vi "ScrumCollection.vi"() -> ()   [LabVIEW 2016]
panel:
  in  "Tab Control":T1(tab)
  out "Summed Signal":dynamicdata(graph)
  out "Maximum Force":dbl
  in  "Tab Control 2":enum32{"Data Collection", "Settings"}(tab)
  out "Collecting?":bool
  in  "Start/Stop Collection":bool
  in  "Reset Graphs":bool
  in  "Pause datastream":bool=TRUE caption="Enable"
  in  "Load Cell 7":bool
  in  "Load Cell 6":bool
  in  "Load Cell 5":bool
  in  "Load Cell 4":bool
  in  "Load Cell 3":bool
  in  "Load Cell 2":bool
  in  "Load Cell 1":bool
  in  "Load Cell 0":bool
  in  "Are you collecting data?":bool
  out "Collected Section":dynamicdata(graph) caption="Section"
  out "Mean Value for last 20 sec":dbl format="%#.6g"
  in  "Load Cell Offset":dbl
  out "Cell 1":dynamicdata(graph)
  out "Cell 0":dynamicdata(graph)
  in  "Load Cell Offset 1":dbl
  out "Mean Value for last 20 sec 1":dbl format="%#.6g"
  out "Cell 2":dynamicdata(graph)
  out "Cell 3":dynamicdata(graph)
  in  "Load Cell Offset 2":dbl
  in  "Load Cell Offset 3":dbl
  out "Mean Value for last 20 sec 2":dbl format="%#.6g"
  out "Mean Value for last 20 sec 3":dbl format="%#.6g"
  out "Cell 4":dynamicdata(graph)
  out "Cell 5":dynamicdata(graph)
  in  "Load Cell Offset 4":dbl
  in  "Load Cell Offset 5":dbl
  out "Mean Value for last 20 sec 4":dbl format="%#.6g"
  out "Mean Value for last 20 sec 5":dbl format="%#.6g"
  out "Cell 6":dynamicdata(graph)
  out "Cell 7":dynamicdata(graph)
  in  "Load Cell Offset 6":dbl
  in  "Load Cell Offset 7":dbl
  out "Mean Value for last 20 sec 6":dbl format="%#.6g"
  out "Mean Value for last 20 sec 7":dbl format="%#.6g"
  out "Balance":dbl(knob) scale=-2000.0..2000.0
  in  "stop":bool
  # "Which load cells should be included in the main graph?"
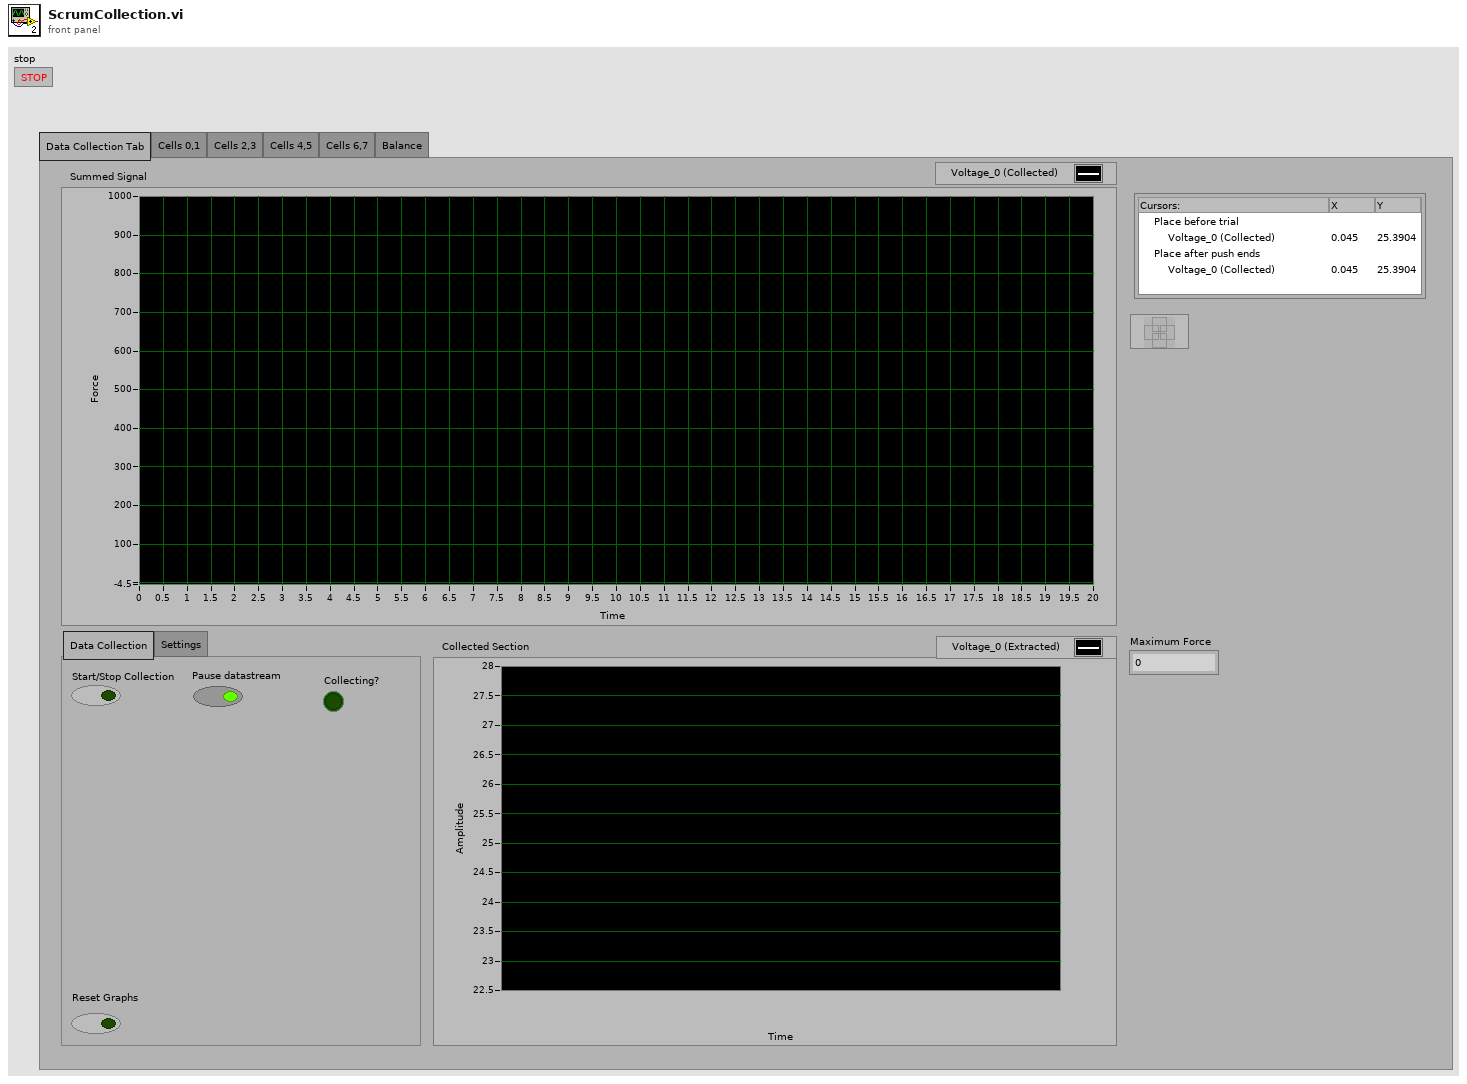
[diagram p1: front panel]
types:
  T1 = enum32{"Data Collection Tab", "Cells 0,1", "Cells 2,3", "Cells 4,5", "Cells 6,7", "Balance"}
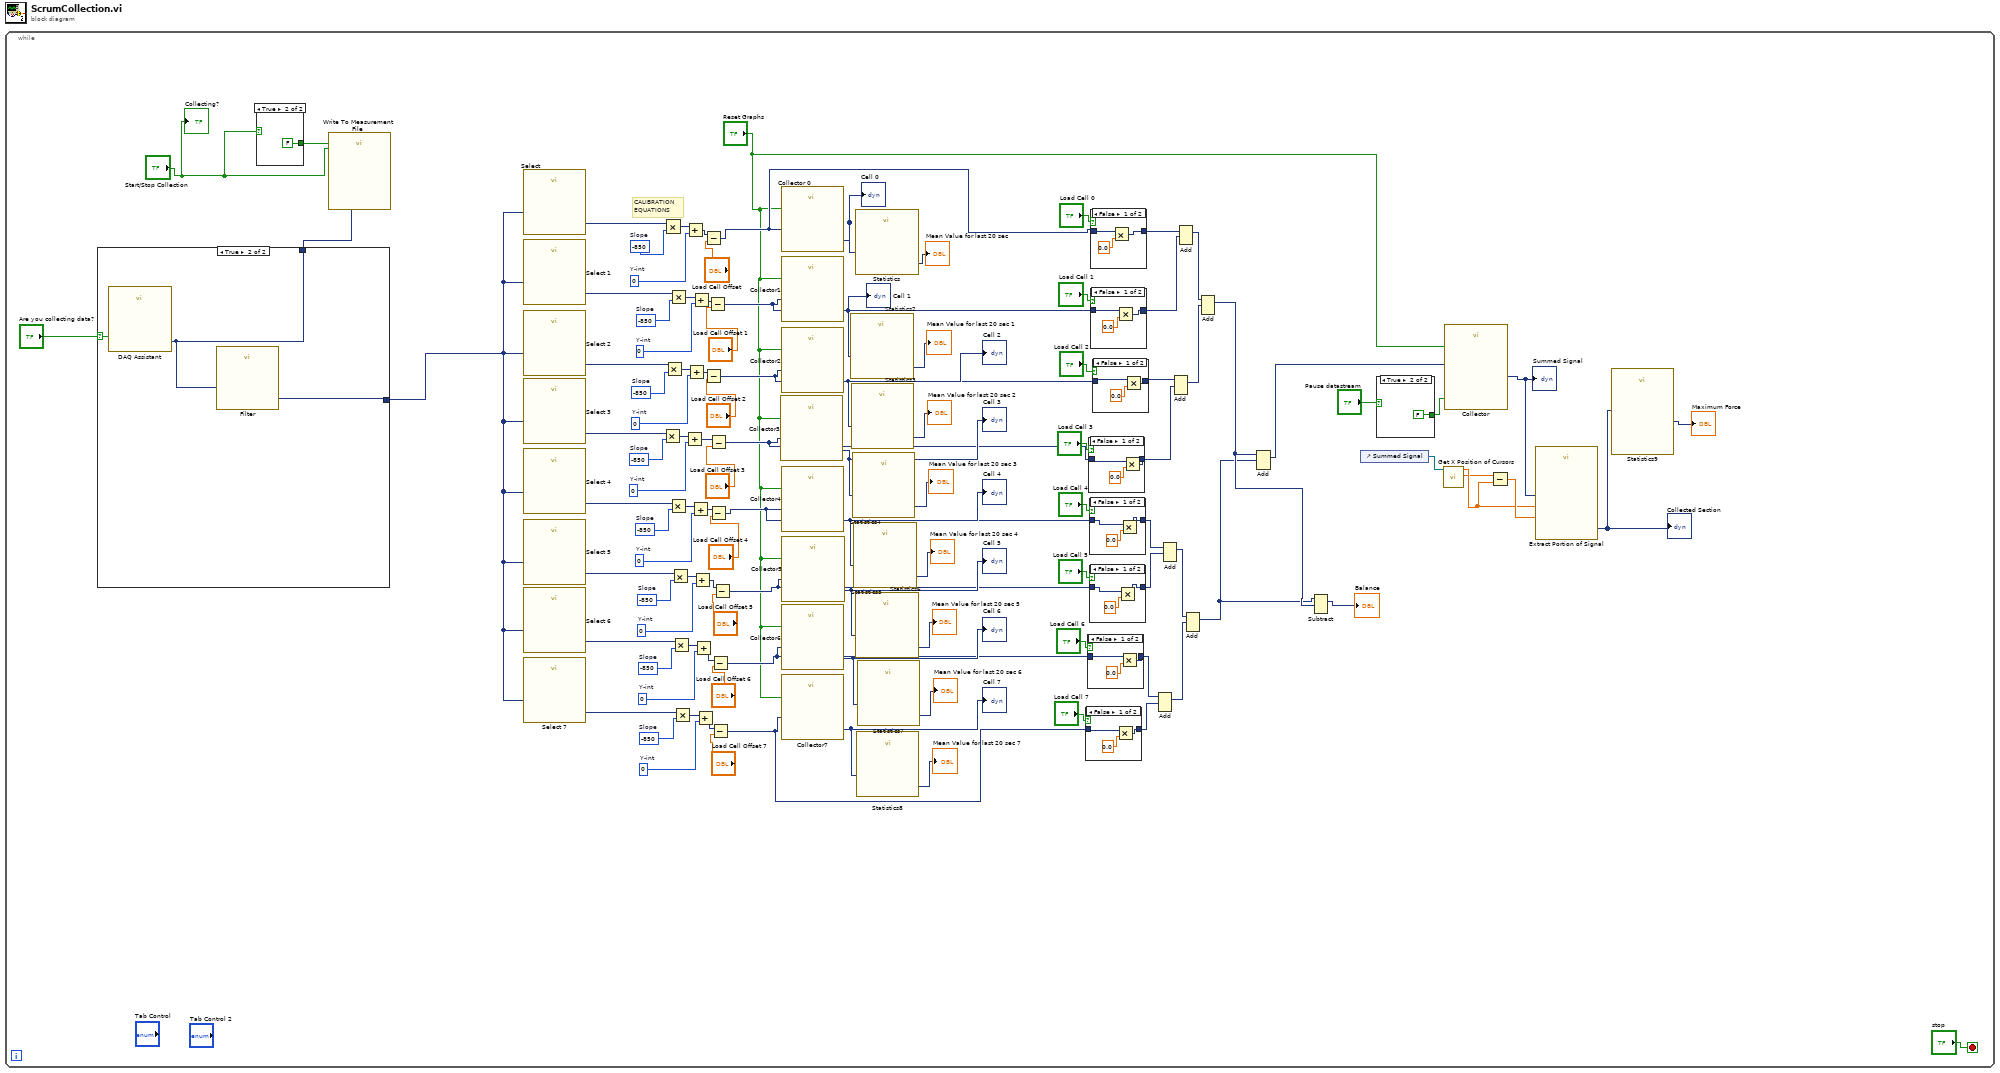
[diagram p0: block diagram]
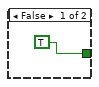
[diagram p2: hidden frame]
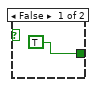
[diagram p3: hidden frame]
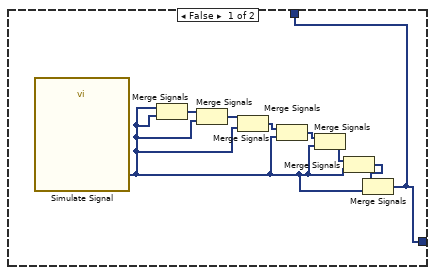
[diagram p4: hidden frame]
diagram:
  n1 = while {
    stop <- "stop" stop-if-true
    w56 = -850  # Slope
    w89 = 0  # Y-int
    w91 = -850  # Slope
    w92 = 0  # Y-int
    w94 = -850  # Slope
    w95 = 0  # Y-int
    w97 = -850  # Slope
    w98 = 0  # Y-int
    w100 = -850  # Slope
    w101 = 0  # Y-int
    w103 = -850  # Slope
    w104 = 0  # Y-int
    w106 = -850  # Slope
    w107 = 0  # Y-int
    w109 = -850  # Slope
    w110 = 0  # Y-int
    # "CALIBRATION\nEQUATIONS"
    n2 = case shown="True" "Are you collecting data?" {
      tunnel: [w117 w126] -> w38
      tunnel: [w117 w125] -> w33
      frame False {
        n3 = call "Simulate Signal"() -> ("Sine with Uniform Noise"=w124:dynamicdata)  [unwired: 14 in, 1 out]
        n4 = Merge Signals(w124, w124) -> (w118:dynamicdata)
        n5 = Merge Signals(w118, w124) -> (w119:dynamicdata)
        n6 = Merge Signals(w119, w124) -> (w120:dynamicdata)
        n7 = Merge Signals(w120, w124) -> (w121:dynamicdata)
        n8 = Merge Signals(w121, w124) -> (w122:dynamicdata)
        n9 = Merge Signals(w122, w124) -> (w123:dynamicdata)
        n10 = Merge Signals(w123, w124) -> (w117:dynamicdata)
      }
      frame True {
        n11 = call "DAQ Assistant"() -> ("data"=w125:dynamicdata)  [unwired: 17 in, 2 out]
        n12 = call "Filter"("Signal"=w125) -> ("Filtered Signal"=w126:dynamicdata)  [unwired: 9 in, 1 out]
      }
    }
    n13 = case shown="True" "Start/Stop Collection" {
      tunnel: [TRUE FALSE] -> w19
      frame False {
      }
      frame True {
      }
    }
    n14 = call "Write To Measurement File"("Signals"=w33, "Reset"=w19, "Enable"="Start/Stop Collection") -> ()  [unwired: 14 in, 3 out]
    n15 = call "Select"("Signals"=w38) -> ("Signal Out"=w57:dynamicdata)  [unwired: 9 in, 1 out]
    n16 = call "Select 1"("Signals"=w38) -> ("Signal Out"=w88:dynamicdata)  [unwired: 9 in, 1 out]
    n17 = call "Select 2"("Signals"=w38) -> ("Signal Out"=w87:dynamicdata)  [unwired: 9 in, 1 out]
    n18 = call "Select 3"("Signals"=w38) -> ("Signal Out"=w86:dynamicdata)  [unwired: 9 in, 1 out]
    n19 = call "Select 4"("Signals"=w38) -> ("Signal Out"=w85:dynamicdata)  [unwired: 9 in, 1 out]
    n20 = call "Select 5"("Signals"=w38) -> ("Signal Out"=w84:dynamicdata)  [unwired: 9 in, 1 out]
    n21 = call "Select 6"("Signals"=w38) -> ("Signal Out"=w83:dynamicdata)  [unwired: 9 in, 1 out]
    n22 = call "Select 7"("Signals"=w38) -> ("Signal Out"=w82:dynamicdata)  [unwired: 9 in, 1 out]
    n23 = Multiply(x=w86, y=w103) -> (x*y=w102:dynamicdata)
    n24 = Multiply(x=w57, y=w56) -> (x*y=w111:dynamicdata)
    n25 = Multiply(x=w87, y=w106) -> (x*y=w105:dynamicdata)
    n26 = Multiply(x=w85, y=w100) -> (x*y=w99:dynamicdata)
    n27 = Multiply(x=w88, y=w109) -> (x*y=w108:dynamicdata)
    n28 = Multiply(x=w84, y=w97) -> (x*y=w96:dynamicdata)
    n29 = Multiply(x=w83, y=w94) -> (x*y=w93:dynamicdata)
    n30 = Multiply(x=w82, y=w91) -> (x*y=w90:dynamicdata)
    n31 = Add(x=w102, y=w101) -> (x+y=w73:dynamicdata)
    n32 = Add(x=w111, y=w110) -> (x+y=w81:dynamicdata)
    n33 = Add(x=w105, y=w104) -> (x+y=w75:dynamicdata)
    n34 = Add(x=w99, y=w98) -> (x+y=w72:dynamicdata)
    n35 = Add(x=w108, y=w107) -> (x+y=w77:dynamicdata)
    n36 = Add(x=w96, y=w95) -> (x+y=w70:dynamicdata)
    n37 = Add(x=w93, y=w92) -> (x+y=w68:dynamicdata)
    n38 = Add(x=w90, y=w89) -> (x+y=w66:dynamicdata)
    n39 = Subtract(x=w81, y="Load Cell Offset") -> (x-y=w31:dynamicdata)
    n40 = Subtract(x=w75, y="Load Cell Offset 2") -> (x-y=w29:dynamicdata)
    n41 = Subtract(x=w77, y="Load Cell Offset 1") -> (x-y=w30:dynamicdata)
    n42 = Subtract(x=w72, y="Load Cell Offset 4") -> (x-y=w27:dynamicdata)
    n43 = Subtract(x=w73, y="Load Cell Offset 3") -> (x-y=w28:dynamicdata)
    n44 = Subtract(x=w68, y="Load Cell Offset 6") -> (x-y=w25:dynamicdata)
    n45 = Subtract(x=w66, y="Load Cell Offset 7") -> (x-y=w24:dynamicdata)
    n46 = Subtract(x=w70, y="Load Cell Offset 5") -> (x-y=w26:dynamicdata)
    n47 = call "Collector3"("Reset"="Reset Graphs", "Signals"=w28) -> ("Collected Signals"=w48:dynamicdata)  [unwired: 8 in, 1 out]
    "Cell 3" <- w48
    n48 = call "Collector 0"("Reset"="Reset Graphs", "Signals"=w31) -> ("Collected Signals"=w54:dynamicdata)  [unwired: 8 in, 1 out]
    "Cell 0" <- w54
    n49 = call "Collector1"("Reset"="Reset Graphs", "Signals"=w30) -> ("Collected Signals"=w52:dynamicdata)  [unwired: 8 in, 1 out]
    "Cell 1" <- w52
    n50 = call "Collector2"("Reset"="Reset Graphs", "Signals"=w29) -> ("Collected Signals"=w50:dynamicdata)  [unwired: 8 in, 1 out]
    "Cell 2" <- w50
    n51 = call "Collector4"("Reset"="Reset Graphs", "Signals"=w27) -> ("Collected Signals"=w46:dynamicdata)  [unwired: 8 in, 1 out]
    "Cell 4" <- w46
    n52 = call "Collector6"("Reset"="Reset Graphs", "Signals"=w25) -> ("Collected Signals"=w41:dynamicdata)  [unwired: 8 in, 1 out]
    "Cell 6" <- w41
    n53 = call "Collector7"("Reset"="Reset Graphs", "Signals"=w24) -> ("Collected Signals"=w40:dynamicdata)  [unwired: 8 in, 1 out]
    "Cell 7" <- w40
    n54 = call "Collector5"("Reset"="Reset Graphs", "Signals"=w26) -> ("Collected Signals"=w42:dynamicdata)  [unwired: 8 in, 1 out]
    "Cell 5" <- w42
    n55 = call "Statistics2"("Signals"=w52) -> ("Arithmetic Mean"=→"Mean Value for last 20 sec 1":dynamicdata)  [unwired: 25 in, 1 out]
    n56 = call "Statistics3"("Signals"=w50) -> ("Arithmetic Mean"=→"Mean Value for last 20 sec 2":dynamicdata)  [unwired: 25 in, 1 out]
    n57 = call "Statistics4"("Signals"=w48) -> ("Arithmetic Mean"=→"Mean Value for last 20 sec 3":dynamicdata)  [unwired: 25 in, 1 out]
    n58 = call "Statistics5"("Signals"=w46) -> ("Arithmetic Mean"=→"Mean Value for last 20 sec 4":dynamicdata)  [unwired: 25 in, 1 out]
    n59 = call "Statistics"("Signals"=w54) -> ("Arithmetic Mean"=→"Mean Value for last 20 sec":dynamicdata)  [unwired: 25 in, 1 out]
    n60 = call "Statistics6"("Signals"=w42) -> ("Arithmetic Mean"=→"Mean Value for last 20 sec 5":dynamicdata)  [unwired: 25 in, 1 out]
    n61 = call "Statistics8"("Signals"=w40) -> ("Arithmetic Mean"=→"Mean Value for last 20 sec 7":dynamicdata)  [unwired: 25 in, 1 out]
    n62 = call "Statistics7"("Signals"=w41) -> ("Arithmetic Mean"=→"Mean Value for last 20 sec 6":dynamicdata)  [unwired: 25 in, 1 out]
    n63 = case shown="False" "Load Cell 7" {
      tunnel: w24 -> [w127 w130]
      tunnel: [w128 w130] -> w13
      frame False {
        n64 = Multiply(x=w127, y=0.0) -> (x*y=w128:dynamicdata)
      }
      frame True {
      }
    }
    n65 = case shown="False" "Load Cell 6" {
      tunnel: [w132 w134] -> w14
      tunnel: w25 -> [w131 w134]
      frame False {
        n66 = Multiply(x=w131, y=0.0) -> (x*y=w132:dynamicdata)
      }
      frame True {
      }
    }
    n67 = case shown="False" "Load Cell 3" {
      tunnel: w28 -> [w144 w146]
      tunnel: [w143 w146] -> w5
      frame False {
        n68 = Multiply(x=w144, y=0.0) -> (x*y=w143:dynamicdata)
      }
      frame True {
      }
    }
    n69 = case shown="False" "Load Cell 4" {
      tunnel: w27 -> [w140 w142]
      tunnel: [w139 w142] -> w16
      frame False {
        n70 = Multiply(x=w140, y=0.0) -> (x*y=w139:dynamicdata)
      }
      frame True {
      }
    }
    n71 = case shown="False" "Load Cell 5" {
      tunnel: w26 -> [w136 w138]
      tunnel: [w135 w138] -> w15
      frame False {
        n72 = Multiply(x=w136, y=0.0) -> (x*y=w135:dynamicdata)
      }
      frame True {
      }
    }
    n73 = case shown="False" "Load Cell 1" {
      tunnel: [w152 w154] -> w7
      tunnel: w30 -> [w151 w154]
      frame False {
        n74 = Multiply(x=w151, y=0.0) -> (x*y=w152:dynamicdata)
      }
      frame True {
      }
    }
    n75 = case shown="False" "Load Cell 0" {
      tunnel: w31 -> [w156 w158]
      tunnel: [w155 w158] -> w8
      frame False {
        n76 = Multiply(x=w156, y=0.0) -> (x*y=w155:dynamicdata)
      }
      frame True {
      }
    }
    n77 = case shown="False" "Load Cell 2" {
      tunnel: w29 -> [w148 w150]
      tunnel: [w147 w150] -> w6
      frame False {
        n78 = Multiply(x=w148, y=0.0) -> (x*y=w147:dynamicdata)
      }
      frame True {
      }
    }
    n79 = Add(1:w13, 2:w14) -> (0:w12:dynamicdata)  [unwired: 1 in, 1 out]
    n80 = Add(1:w15, 2:w16) -> (0:w11:dynamicdata)  [unwired: 1 in, 1 out]
    n81 = Add(1:w5, 2:w6) -> (0:w10:dynamicdata)  [unwired: 1 in, 1 out]
    n82 = Add(1:w7, 2:w8) -> (0:w9:dynamicdata)  [unwired: 1 in, 1 out]
    n83 = Add(1:w12, 2:w11) -> (0:w1:dynamicdata)  [unwired: 1 in, 1 out]
    n84 = Add(1:w10, 2:w9) -> (0:w2:dynamicdata)  [unwired: 1 in, 1 out]
    n85 = Add(1:w1, 2:w2) -> (0:w4:dynamicdata)  [unwired: 1 in, 1 out]
    n86 = Subtract(1:w2, 2:w1) -> (0:→"Balance":dynamicdata)  [unwired: 1 in, 1 out]
    n87 = control-ref of="Summed Signal"() -> (w36:refnum<vi>)
    n88 = case shown="True" "Pause datastream" {
      tunnel: [TRUE FALSE] -> w17
      frame False {
      }
      frame True {
      }
    }
    n89 = call "Get X Position of Cursors.vi"("WaveformGraph in"=w36) -> ("Cursor 2 X Pos"=w34:dbl, "Cursor 1 X Pos"=w35:dbl)  [unwired: 7 in, 1 out]
    n90 = call "Collector"("Reset"="Reset Graphs", "Enable"=w17, "Signals"=w4) -> ("Collected Signals"=w32:dynamicdata)  [unwired: 7 in, 1 out]
    "Summed Signal" <- w32
    n91 = Subtract(x=w34, y=w35) -> (x-y=w37:dbl)
    n92 = call "Extract Portion of Signal"("Length"=w37, "Begin Offset"=w35, "Signals"=w32) -> ("Section"=w21:dynamicdata)  [unwired: 7 in, 1 out]
    "Collected Section" <- w21
    n93 = call "Statistics9"("Signals"=w21) -> ("Maximum"=→"Maximum Force":dynamicdata)  [unwired: 25 in, 1 out]
    "Collecting?" <- "Start/Stop Collection"
  }
